vi "Delete All Subsystems in Tree.vi"(8 "error in (no error)":errorcluster, 11 "Tree Control":refnum<vi>) -> (0 "error out":errorcluster, 3 "dup Tree Control":refnum<vi>)   [LabVIEW 2024]
doc: "Deletes all the subsystems in the tree control."
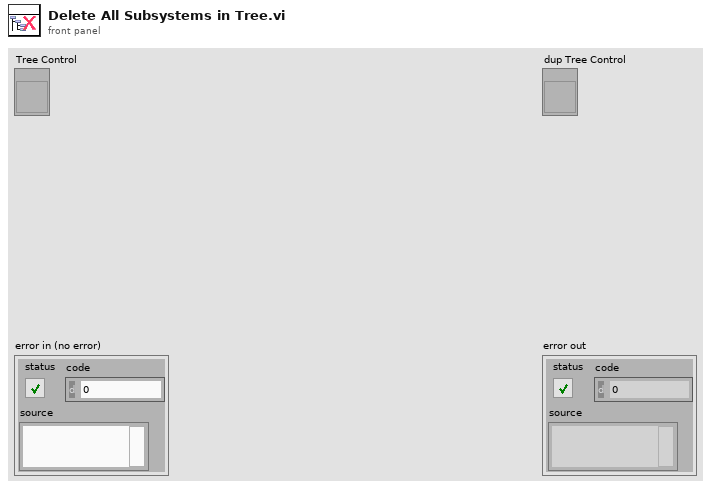
[diagram p1: front panel]
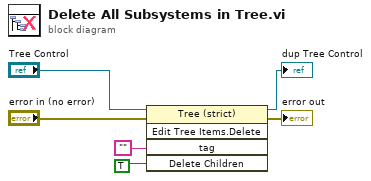
[diagram p0: block diagram]
diagram:
  n1 = invoke class="Tree (strict)" method="Edit Tree Items.Delete"(reference="Tree Control", error in="error in (no error)", "tag"="" ("Tag"), "Delete Children"=TRUE ("Delete Children?")) -> (reference out=→"dup Tree Control":refnum<vi>, error out=→"error out":errorcluster)  [unwired: 1 in, 3 out]
